vi "Is Array Constant.vi"(1 "Array":dbl[](array[numeric])) -> (0 "is constant?":bool)   [LabVIEW 2015]
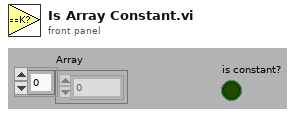
[diagram p1: front panel]
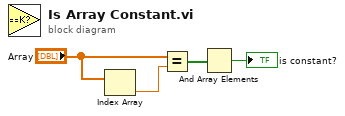
[diagram p0: block diagram]
diagram:
  n1 = Index Array(array="Array") -> (element=w4:dbl)  [unwired: 1 in]
  n2 = Equal?(x="Array", y=w4) -> (x = y?=w2:bool[])
  n3 = And Array Elements(Boolean array=w2) -> (logical AND=→"is constant?":bool)
